vi "Extended Image To Image.vi"(11 "Extended Image":T2) -> (3 "Image":T1)   [LabVIEW 2020, in "G-Image.lvlib"]
doc: "Convert the extended image to a LabVIEW image. Extracts the first frame of an animated gif and discards the rest."
uses:
  G-Image.lvlib
  Extended Image.ctl
  <vilib>/picture/picture.llb/imagedata.ctl
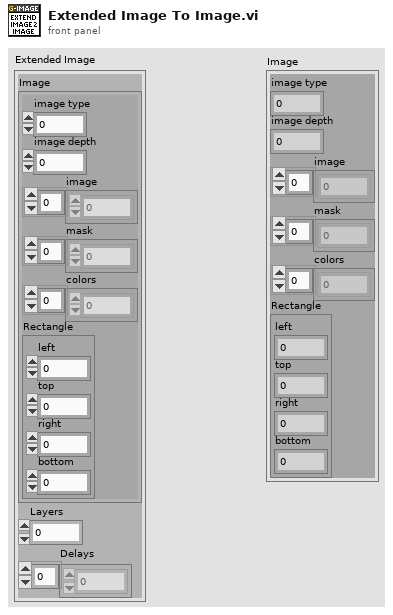
[diagram p1: front panel]
types:
  T1 = typedef "imagedata.ctl" = cluster{"image type":i32, "image depth":i32, "image":u8[], "mask":u8[], "colors":u32[], "Rectangle":cluster{"left":i16, "top":i16, "right":i16, "bottom":i16}}
  T2 = typedef "G-Image.lvlib/Extended Image.ctl" = cluster{"Image":T1, "Layers":i32, "Delays":i32[]}
  T3 = cluster{"left":i16, "top":i16, "right":i16, "bottom":i16}
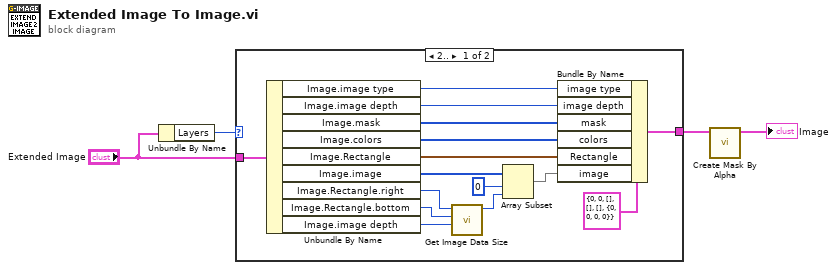
[diagram p0: block diagram]
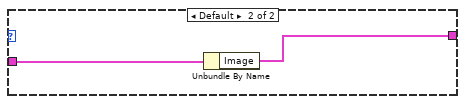
[diagram p2: hidden frame]
diagram:
  n1 = Unbundle By Name("Extended Image") -> ("Layers"=w4:i32)
  n2 = case shown="2.." w4 {
    tunnel: "Extended Image" -> [w10 w21]
    tunnel: [w9 w20] -> w1
    frame 2.. {
      n3 = Unbundle By Name(w10) -> ("Image.image type"=w13:i32, "Image.image depth"=w14:i32, "Image.mask"=w15:u8[], "Image.colors"=w16:u32[], "Image.Rectangle"=w17:T3, "Image.image"=w11:u8[], "Image.Rectangle.right"=w8:i16, "Image.Rectangle.bottom"=w7:i16, "Image.image depth"=w6:i32)
      n4 = call "Get Image Data Size.vi"("Depth"=w6, "Height"=w7, "Width"=w8) -> ("Image Data Size"=w5:i32)  [unwired: 8 in]
      n5 = Array Subset(array=w11, index=0, length=w5) -> (w18:u8[])
      n6 = Bundle By Name(cluster=T1 {"image type"=0, "image depth"=0, "image"=[], "mask"=[], "colors"=[], "Rectangle"={"left"=0, "top"=0, "right"=0, "bottom"=0}} ("masked image data"), "image type"=w13, "image depth"=w14, "mask"=w15, "colors"=w16, "Rectangle"=w17, "image"=w18) -> (w9:T1)
    }
    frame Default {
      n7 = Unbundle By Name(w21) -> ("Image"=w20:T1)
    }
  }
  n8 = call <vilib>:"Create Mask By Alpha.vi"("image data"=w1) -> ("masked image data"=→"Image":T1)  [unwired: 10 in]
